vi "UsrProfiles-Remove user name prefix.vi"(11 "Profile name (full)":string) -> (2 "Profile name (user removed)":string)   [LabVIEW 2020]
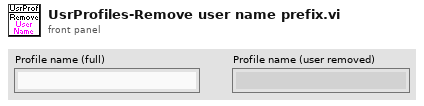
[diagram p1: front panel]
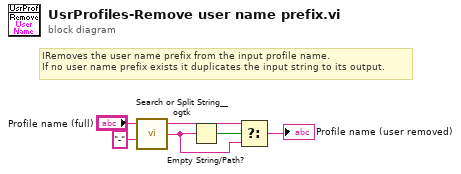
[diagram p0: block diagram]
diagram:
  # "IRemoves the user name prefix from the input profile name.\nIf no user name prefix exists it duplicates the input string to its output."
  n1 = call <userlib>:"Search or Split String__ogtk.vi"("search string/char (-)"="-", "string"="Profile name (full)") -> ("substring after match"=w2:string, "substring before match"=w3:string)  [unwired: 1 in, 1 out]
  n2 = Empty String/Path?(string/path=w2) -> (empty?=w4:bool)
  n3 = Select(t=w3, s=w4, f=w2) -> (s? t:f=→"Profile name (user removed)":string)
